vi "Actor Core.vi"(8 "error in":errorcluster, 11 "Sender Loop in":refnum<class "Sender Loop.lvclass">) -> (0 "error out":errorcluster, 3 "Actor out":refnum<class "Actor.lvclass">)   [LabVIEW 2021, in "Secure Echo Broadcast Test Server Manager.lvlib" / "Sender Loop.lvclass"]
doc: "(<B>Filename</B>: Actor Framework.lvlib:Actor.lvclass:Actor Core.vi)\n\nReceives messages to the actor, reacts to them, and initiates any error handling that may shut the actor down.\n\nDescendant classes may override this VI to append parallel tasks for the actor to complete while it handles messages. Overrides use the Call Parent Method node."
uses:
  Sender Loop.lvclass
  C:/Program Files/National Instruments/LabVIEW 2021/vi.lib/ActorFramework/Actor/Actor.lvclass
  <vilib>/ActorFramework/Actor/Actor.lvclass
  <vilib>/ActorFramework/Actor/Actor.lvclass/Actor.ctl
  <vilib>/ActorFramework/Message Enqueuer/Message Enqueuer.lvclass/Message Enqueuer.ctl
  Sender Loop.lvclass/Sender Loop.ctl
  <vilib>/ActorFramework/Message Enqueuer/Init from Existing Queue.vi
  <vilib>/ActorFramework/Message Enqueuer/Enqueue.vi
  <vilib>/ActorFramework/Stop Msg/Stop Msg.lvclass
  C:/Program Files/National Instruments/LabVIEW 2021/vi.lib/ActorFramework/Message/Message.lvclass
  <vilib>/Utility/LVClass/Get LV Class Name.vi
  <resource>/AFDebug/Generate Trace for Message.vi
  <vilib>/ActorFramework/Message Priority Queue/Priority Enqueue.vi
  <vilib>/ActorFramework/Message Enqueuer/Message Enqueuer.lvclass
  WebSocket Actor/WebSocket Service Messages/Broadcast Msg/Broadcast Msg.lvclass
  <userlib>/_OpenG.lib/error/error.llb/openg_error.lvlib
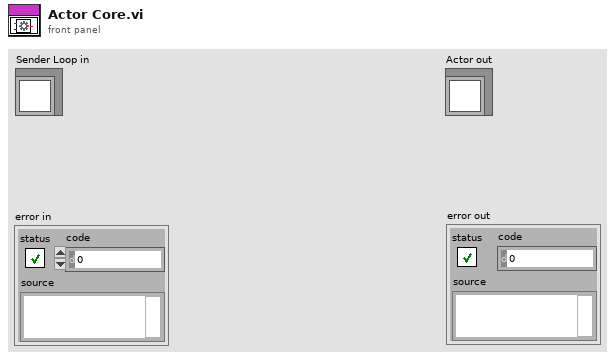
[diagram p1: front panel]
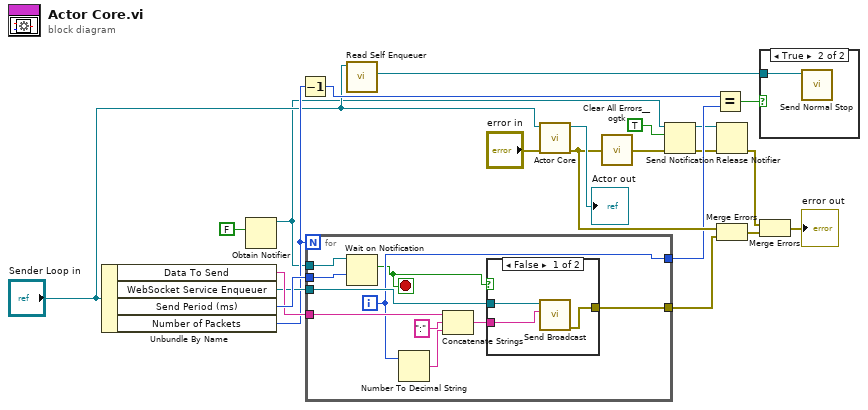
[diagram p0: block diagram]
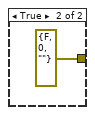
[diagram p3: hidden frame]
diagram:
  n1 = Unbundle By Name("Sender Loop in") -> ("Data To Send"=w18:string, "WebSocket Service Enqueuer"=w17:refnum<class "Message Enqueuer.lvclass">, "Send Period (ms)"=w19:i32, "Number of Packets"=w12:i32)
  n2 = Obtain Notifier(notification data type=FALSE) -> (notifier out=w6:refnum<notifier>)  [unwired: 3 in, 2 out]
  n3 = Decrement(x=w12) -> (x-1=w11:i32)
  n4 = for {
    N: w12 -> [_]
    tunnel: w6 -> [w32]
    tunnel: w19 -> [w31]
    tunnel: w18 -> [w30]
    tunnel: w17 -> [w29]
    tunnel: [w24] -> w13
    tunnel: [w25] -> w7
    i -> [w24]
    stop <- w23 stop-if-true
    n5 = Wait on Notification(notifier=w32, timeout in ms (-1)=w31) -> (notification=w23:bool)  [unwired: 2 in, 3 out]
    n6 = Number To Decimal String(number=w24) -> (decimal integer string=w26:string)  [unwired: 1 in]
    n7 = Concatenate Strings(w30, ":" ("string"), w26) -> (w28:string)
    n8 = case shown="False" w23 {
      tunnel: w29 -> [w35 _]
      tunnel: w28 -> [w34 _]
      tunnel: [w33 errorcluster {"status"=FALSE, "code"=0, "source"=""} ("error out")] -> w25
      frame False {
        n9 = call "Send Broadcast.vi"("Data"=w34, "Message Enqueuer in"=w35) -> ("error out"=w33:errorcluster)  [unwired: 8 in, 1 out]
      }
      frame True {
      }
    }
  }
  n10 = call <vilib>:"Read Self Enqueuer.vi"("Actor"="Sender Loop in") -> ("Self Enqueuer"=w8:refnum<class "Message Enqueuer.lvclass">)  [unwired: 10 in]
  n11 = call-parent "Actor Core.vi"("error in"="error in", "Actor in"="Sender Loop in") -> ("error out"=w16:errorcluster, "Actor out"=→"Actor out":refnum<class "Actor.lvclass">)  [unwired: 8 in]
  n12 = call <userlib>:"Clear All Errors__ogtk.vi"("Error In"=w16) -> ("Error Out"=w15:errorcluster)  [unwired: 3 in]
  n13 = Send Notification(notification=TRUE, notifier=w6, error in (no error)=w15) -> (notifier out=w4:refnum<notifier>, error out=w5:errorcluster)
  n14 = Equal?(x=w11, y=w13) -> (x = y?=w10:bool)
  n15 = Release Notifier(notifier=w4, error in (no error)=w5) -> (error out=w3:errorcluster)  [unwired: 1 in, 2 out]
  n16 = Merge Errors(w16, w7) -> (w1:errorcluster)
  n17 = case shown="True" w10 {
    tunnel: w8 -> [_ w37]
    frame False {
    }
    frame True {
      n18 = call <vilib>:"Send Normal Stop.vi"("Message Enqueuer"=w37) -> ()  [unwired: 10 in, 1 out]
    }
  }
  n19 = Merge Errors(w3, w1) -> (→"error out":errorcluster)
